vi "mqttTXdataQueue.vi"(2 "function":T1=enum."getQueue", 7 "telegram":u8[](array[numeric]), 11 "error in (no error)":errorcluster) -> (4 "Queue out":refnum<queue>, 15 "error out":errorcluster)   [LabVIEW 2013]
uses:
  mqttTXdataQueueFunction.ctl
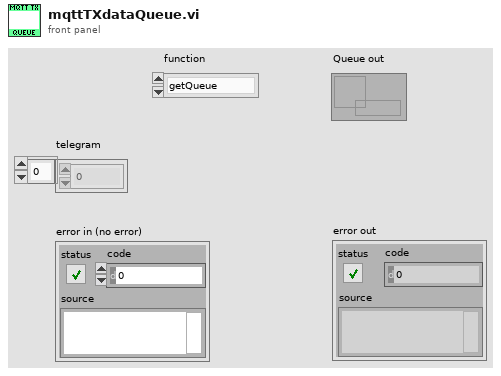
[diagram p1: front panel]
types:
  T1 = typedef "mqttTXdataQueueFunction.ctl" = enum16{"init", "deinit", "getQueue", "enqueue"}
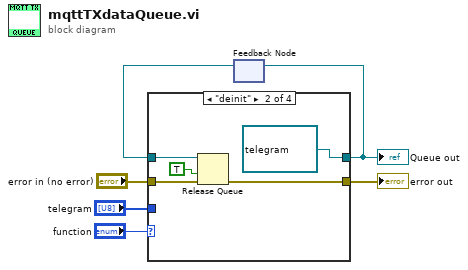
[diagram p0: block diagram]
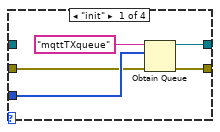
[diagram p2: hidden frame]
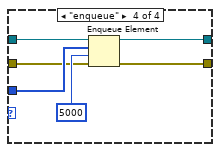
[diagram p4: hidden frame]
diagram:
  n1 = feedback #1() -> (w3:refnum<queue>)  [unwired: 1 in]
  n2 = case shown="\"deinit\"" "function" {
    tunnel: "telegram" -> [w10 _ _ w22]
    tunnel: [w9 refnum<queue> refnum ("queue out") w18 w23] -> w4
    tunnel: w3 -> [_ w16 w18 w24]
    tunnel: "error in (no error)" -> [w7 w13 w17 w20]
    tunnel: [w8 w12 w17 w19] -> w1
    frame "init" {
      n3 = Obtain Queue(name (unnamed)="mqttTXqueue", element data type=w10, error in (no error)=w7) -> (queue out=w9:refnum<queue>, error out=w8:errorcluster)  [unwired: 2 in, 1 out]
    }
    frame "deinit" {
      n4 = Release Queue(queue=w16, force destroy? (F)=TRUE, error in (no error)=w13) -> (error out=w12:errorcluster)  [unwired: 2 out]
    }
    frame "getQueue" {
    }
    frame "enqueue" {
      n5 = Enqueue Element(queue=w24, element=w22, timeout in ms (-1)=5000, error in (no error)=w20) -> (queue out=w23:refnum<queue>, error out=w19:errorcluster)  [unwired: 1 out]
    }
  }
  "Queue out" <- w4
  "error out" <- w1
  n6 = feedback-in #1(w4) -> ()
